vi "setUp.vi"(8 "error in (no error)":errorcluster, 11 "reference in":refnum<class "Scheduled Logging Loopback.lvclass">) -> (0 "error out":errorcluster, 3 "reference out":refnum<class "Scheduled Logging Loopback.lvclass">)   [LabVIEW 2020, in "Scheduled Logging Loopback.lvclass"]
doc: "setUp runs prior to the test method during test execution. Use this method to initialize any object data required by your tests."
uses:
  Scheduled Logging Loopback.lvclass
  C:/Program Files (x86)/National Instruments/LabVIEW 2020/vi.lib/addons/_JKI Toolkits/VI Tester/TestCase.llb/TestCase.lvclass
  Scheduled Logging Loopback.lvclass/Scheduled Logging Loopback.ctl
  <vilib>/addons/_JKI Toolkits/VI Tester/TestCase.llb/TestCase.lvclass
  niveristand-custom-device-testing-tools/VeriStandTestUtilities/VeriStandTestUtilities.lvlib
  <vilib>/WebDAVClient/NI_WebDAV.lvlib
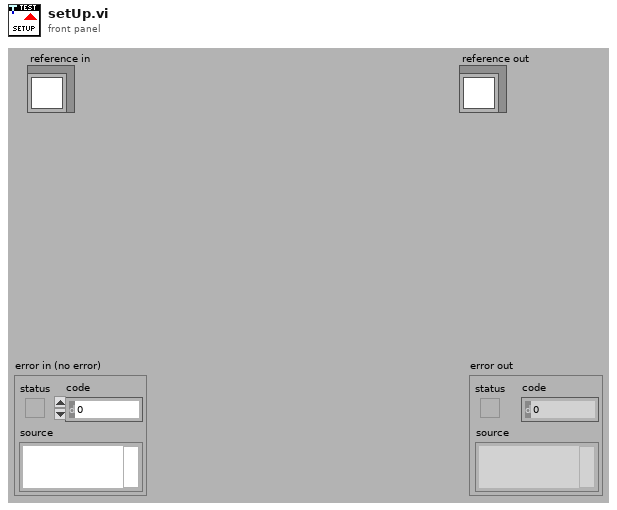
[diagram p1: front panel]
types:
  T1 = typedef "Custom Device API.lvlib/Custom Device Item Ref.ctl" = u64
  T2 = typedef "NI_WebDAV.lvlib/SessionHandle.ctl" = refnum<k1>
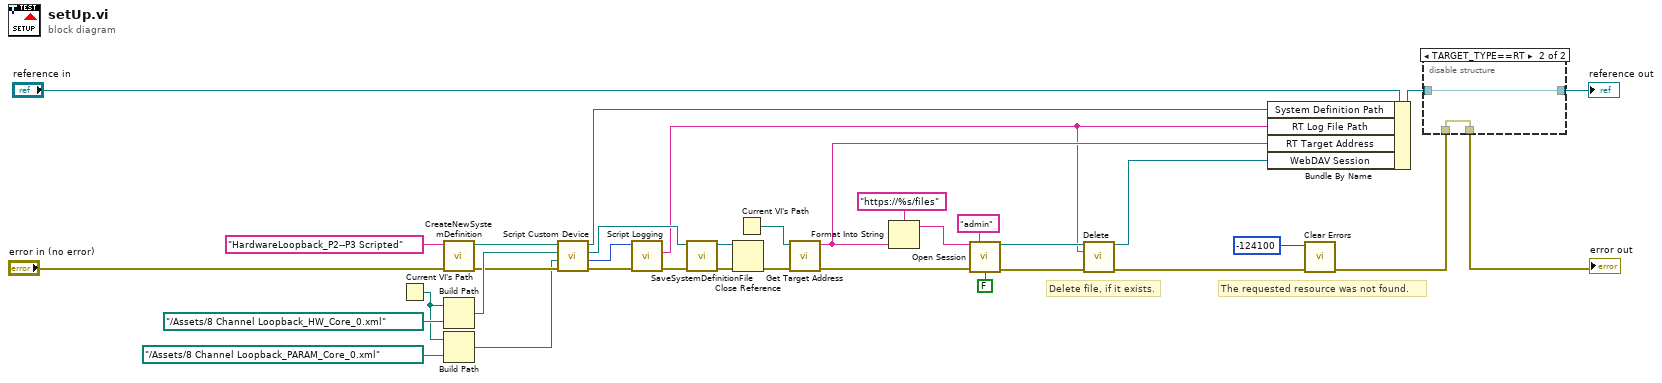
[diagram p0: block diagram]
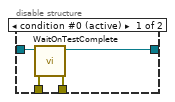
[diagram p2: hidden frame]
diagram:
  # "Delete file, if it exists."
  # "The requested resource was not found."
  n1 = Current VI's Path() -> (path=w16:path)
  n2 = call "CreateNewSystemDefinition.vi"("error in"="error in (no error)", "System Definition Name"="HardwareLoopback_P2--P3 Scripted" ("Channel")) -> ("error out"=w28:errorcluster, "System Definition Path"=w27:path)  [unwired: 8 in]
  n3 = Build Path(base path=w16, name or relative path=path "../Assets/8 Channel Loopback_HW_Core_0.xml" ("Hardware File Path")) -> (appended path=w32:path)
  n4 = Build Path(base path=w16, name or relative path=path "../Assets/8 Channel Loopback_PARAM_Core_0.xml" ("Hardware File Path")) -> (appended path=w17:path)
  n5 = call "Script Custom Device.vi"("error in"=w28, "Parameter File Path"=w17, "Hardware File Path"=w32, "System Definition File Path In"=w27) -> ("error out"=w24:errorcluster, "Ballard ARINC 429 custom device out"=w23:T1, "System Definition Reference"=w26:refnum<k24>, "System Definition File Path Out"=w4:path)  [unwired: 4 in]
  n6 = call "Script Logging.vi"("error in (no error)"=w24, "Ballard ARINC 429 custom device in"=w23) -> ("error out"=w22:errorcluster, "RT log file path"=w8:string)  [unwired: 7 in, 1 out]
  n7 = call "SaveSystemDefinitionFile.vi"("error in (no error)"=w22, "System Definition Reference in"=w26) -> ("error out"=w21:errorcluster, "System Definition Reference out"=w20:refnum<k24>)  [unwired: 8 in]
  n8 = Close Reference(reference=w20, error in (no error)=w21) -> (error out=w18:errorcluster)
  n9 = Current VI's Path() -> (path=w1:path)
  n10 = call "Get Target Address.vi"("error in (no error)"=w18, "calling VI location"=w1) -> ("error out"=w10:errorcluster, "target address"=w9:string)  [unwired: 8 in]
  n11 = Format Into String(format string="https://%s/files" ("host uri prefix"), w9) -> (resulting string=w11:string)  [unwired: 2 in, 1 out]
  n12 = call <vilib>:"Open Session.vi"("host uri prefix"=w11, "username"="admin", "error in (no error)"=w10, "verify server?"=FALSE) -> ("session handle out"=w15:T2, "error out"=w14:errorcluster)  [unwired: 10 in]
  n13 = call <vilib>:"Delete.vi"("session handle"=w15, "relative uri"=w8, "error in (no error)"=w14) -> ("session handle out"=w2:T2, "error out"=w6:errorcluster)  [unwired: 11 in]
  n14 = Bundle By Name(cluster="reference in", "System Definition Path"=w4, "RT Log File Path"=w8, "RT Target Address"=w9, "WebDAV Session"=w2) -> (w19:refnum<class "Scheduled Logging Loopback.lvclass">)
  n15 = call <vilib>:"Clear Errors.vi"("error in (no error)"=w6, "specific error code to clear (0: all)"=-124100) -> ("error out"=w3:errorcluster)  [unwired: 4 in, 1 out]
  n16 = disable-structure shown="TARGET_TYPE==RT" {
    disable-tunnel: w3 -> [w39 w40]
    disable-tunnel: [w38 w40] -> w35
    disable-tunnel: [w37 w41] -> w33
    disable-tunnel: w19 -> [w36 w41]
    frame condition #0 (active) {
      n17 = call <vilib>:"WaitOnTestComplete.vi"("error in (no error)"=w39, "TestCase in"=w36) -> ("error out"=w38:errorcluster, "TestCase out"=w37:refnum<class "Scheduled Logging Loopback.lvclass">)  [unwired: 8 in]
    }
    frame condition #1 {
    }
  }
  "error out" <- w35
  "reference out" <- w33
